vi "subVI REMLAB.vi"(3 "V/div":dbl=1.0, 4 "Scelta server":enum16{"143.225.170.55", "143.225.170.56"}(ring)) -> ()   [LabVIEW 2022 SP3]
panel:
  out "rest of the binary string":string
  out "Control sent":T1(array[cluster])
  in  "Esponente":enum16{"ns", "us", "ms", "s"}(ring)
  in  "Sec a divisione":enum16{"1", "2,5", "5"}(ring)
  out "Frequenza di campionamento":dbl
  out "Segnale scalato":dbl[](graph)
  out "Waveform Graph":i32[](graph)
  out "error out":errorcluster={"status"=TRUE, "code"=63, "source"="TCP Open Connection in main.vi"}
  out "Risposta Server":string[](array[string])
  in  "Control":T1(array[cluster])=[{"Device"=10, "Operation"=0, "Command/byte count"="OUTP:LOAD INF\nAPPL:SIN 1000,10,0"}, {"Device"=1, "Operation"=0, "Command/byte count"="HEAD OFF\nDAT:SOU CH1\nDAT:ENC ASCI\nDAT:WID 1\nDAT:STAR 1\nDAT:STOP 2500\nCH1:SCA 1\nHOR:MAI:SCA 250E-6\nCURV?"}, {"Device"=1, "Operation"=1, "Command/byte count"="15000"}] {"Operation" items=["write", "read"]; "Device" items=["DSO"=1, "AWG"=10]}
  in  "error in (no error)":errorcluster
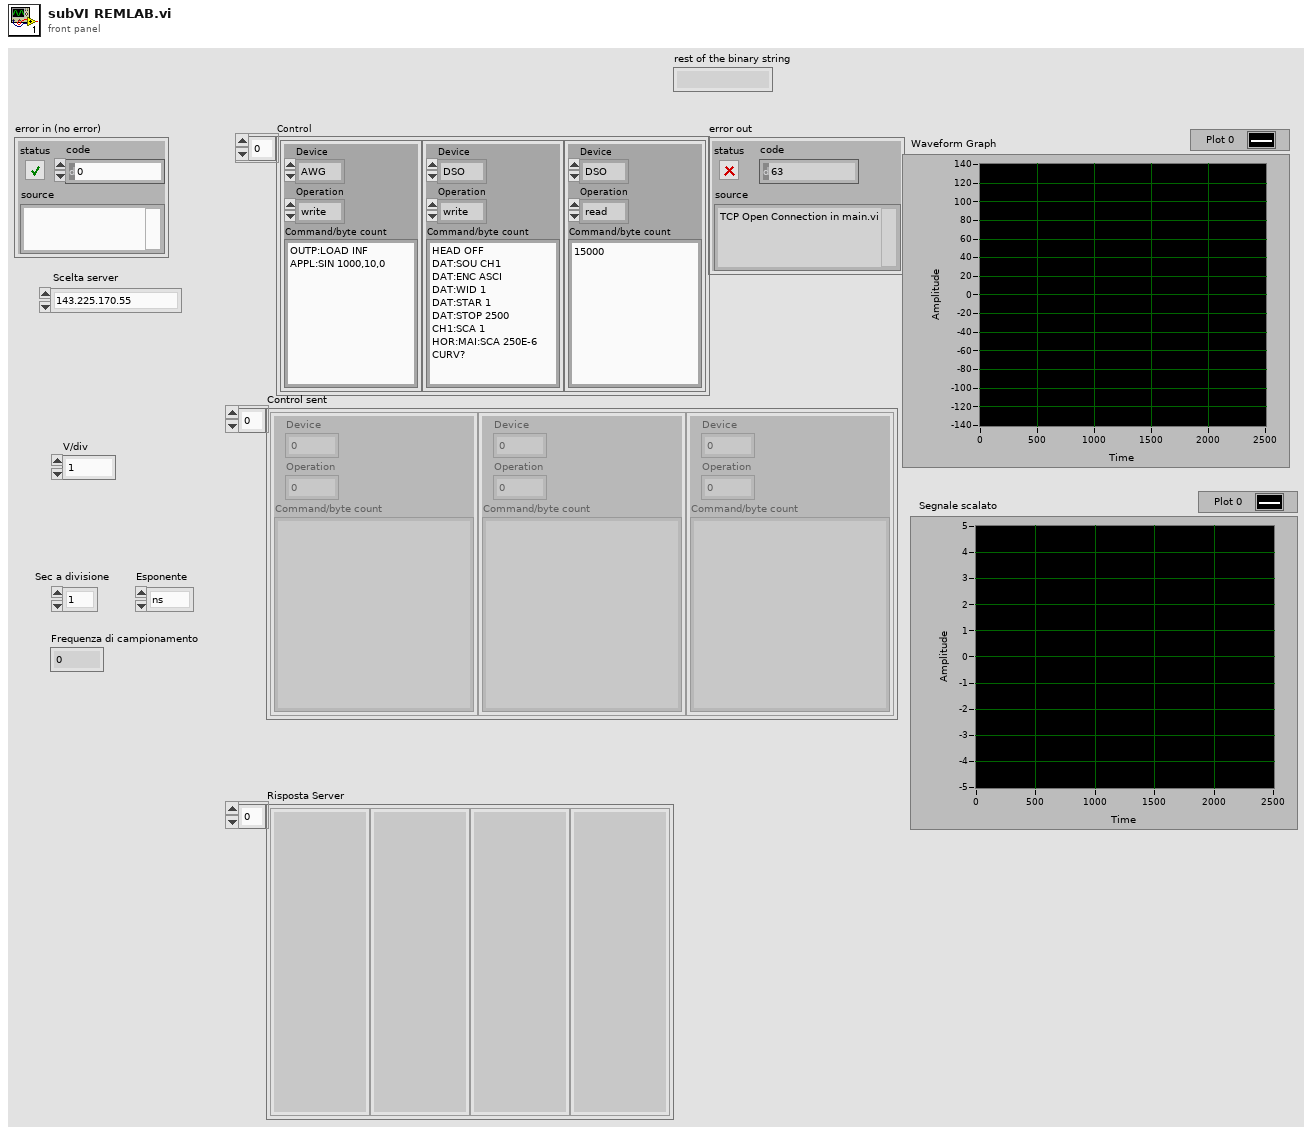
[diagram p1: front panel]
types:
  T1 = cluster{"Device":u16, "Operation":u16, "Command/byte count":string}[]
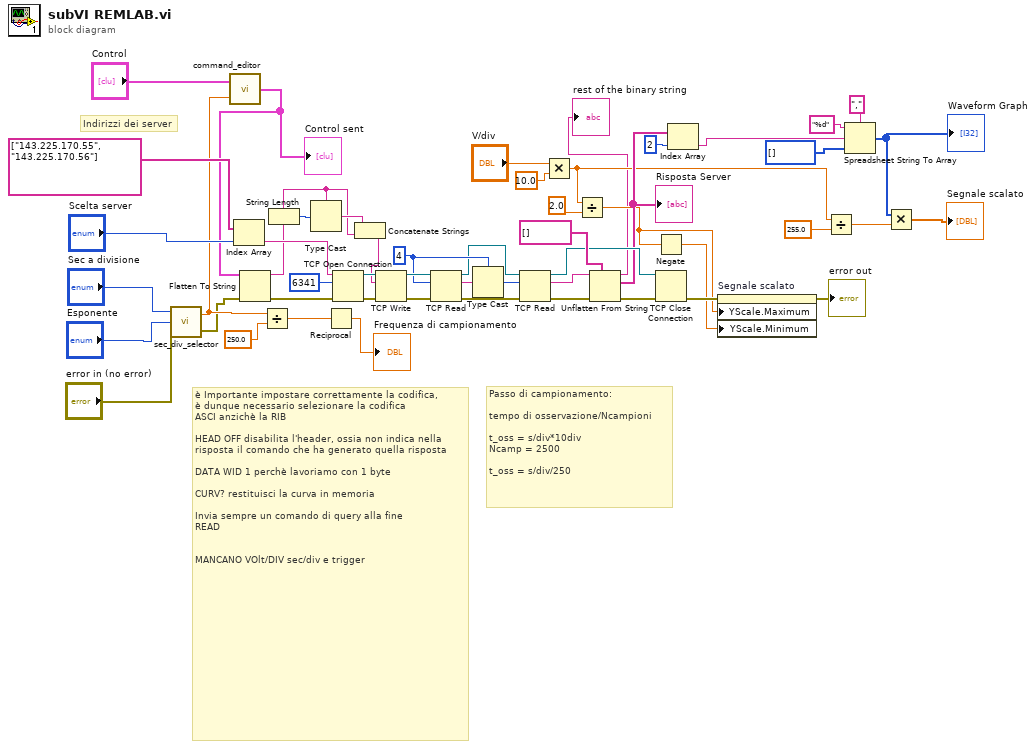
[diagram p0: block diagram]
diagram:
  w43 = 4
  # "Passo di campionamento:\n\ntempo di osservazione/Ncampioni\n\nt_oss = s/div*10div\nNcamp = 2500\n\nt_oss = s/div/250"
  # "è Importante impostare correttamente la codifica,\nè dunque necessario selezionare la codifica \nASCI anzichè la RIB\n\nHEAD OFF disabilita l'header, ossia non indica nella \nrisposta il comando che ha generato quella risposta\n\nDATA WID 1 perchè lavoriamo con 1 byte\n\nCURV? restituisci la curva in memoria\n\nInvia sempre un comando di query alla fine\nREAD\n\n\nMANCANO VOlt/DIV sec/div e trigger"
  # "Indirizzi dei server"
  n1 = call "sec_div_selector.vi"("error in (no error)"="error in (no error)", "Esponente"="Esponente", "Sec a divisione"="Sec a divisione") -> ("error out"=w4:errorcluster, "sec/div"=w5:ext)
  n2 = call "command_editor.vi"("s/div"=w5, "Control"="Control") -> ("output array"=w3:T1)
  "Control sent" <- w3
  n3 = Index Array(array=string[] ["143.225.170.55", "143.225.170.56"], index="Scelta server") -> (element=w50:string)
  n4 = Flatten To String(anything=w3, error in (no error)=w4) -> (data string=w1:string, error out=w11:errorcluster)  [unwired: 2 in, 1 out]
  n5 = Divide(x=w5, y=250.0) -> (x/y=w14:ext)
  n6 = String Length(string=w1) -> (length=w47:i32)
  n7 = Type Cast(type=w1, x=w47) -> (*(type *) &x=w46:string)
  n8 = Reciprocal(x=w14) -> (1/x=→"Frequenza di campionamento":ext)
  n9 = TCP Open Connection(address=w50, remote port or service name=u16 6341, error in (no error)=w11) -> (connection ID=w48:refnum<k5>, error out=w49:errorcluster)  [unwired: 2 in]
  n10 = Concatenate Strings(w46, w1) -> (w36:string)
  n11 = TCP Write(connection ID=w48, data in=w36, error in (no error)=w49) -> (connection ID out=w44:refnum<k5>, error out=w45:errorcluster)  [unwired: 1 in, 1 out]
  n12 = TCP Read(connection ID=w44, bytes to read=w43, error in (no error)=w45) -> (connection ID out=w37:refnum<k5>, data out=w42:string, error out=w40:errorcluster)  [unwired: 2 in]
  n13 = Type Cast(type=w43, x=w42) -> (*(type *) &x=w38:i32)
  n14 = TCP Read(connection ID=w37, bytes to read=w38, error in (no error)=w40) -> (connection ID out=w35:refnum<k5>, data out=w41:string, error out=w34:errorcluster)  [unwired: 2 in]
  n15 = Multiply(x="V/div", y=10.0) -> (x*y=w21:dbl)
  n16 = Divide(x=w21, y=2.0) -> (x/y=w18:dbl)
  n17 = Unflatten From String(type=string[] [] ("String Array"), binary string=w41, error in (no error)=w34) -> (rest of the binary string=→"rest of the binary string":string, value=w32:string[], error out=w33:errorcluster)  [unwired: 2 in]
  "Risposta Server" <- w32
  n18 = Negate(x=w18) -> (-x=w19:dbl)
  n19 = TCP Close Connection(connection ID=w35, error in (no error)=w33) -> (error out=w22:errorcluster)  [unwired: 1 in, 1 out]
  n20 = Index Array(array=w32, index=2) -> (element=w30:string)
  n21 = property on="Segnale scalato" class="WFGraph (strict)"(error in=w22, "YScale.Maximum"=w18, "YScale.Minimum"=w19) -> (error out=→"error out":errorcluster)  [unwired: 1 in, 1 out]
  n22 = Divide(x=w21, y=255.0) -> (x/y=w23:dbl)
  n23 = Spreadsheet String To Array(delimiter (Tab)=",", format string="%d", spreadsheet string=w30, array type (2D Dbl)=i32[] []) -> (array=w13:i32[])
  "Waveform Graph" <- w13
  n24 = Multiply(x=w13, y=w23) -> (x*y=→"Segnale scalato":dbl[])
